vi "sub-select BT device.vi"(8 "error in (no error)":errorcluster, 11 "device list":T1(array[cluster])) -> (0 "error out":errorcluster, 2 "Canceled by user":bool, 3 "Address":string)   [LabVIEW 2016]
doc: "The VI prompts a window that allows the user to select the device and returns the selected device address."
panel:
  in  "Cancel Button":bool
  in  "OK Button":bool
  in  "Select Device":i32(listbox)
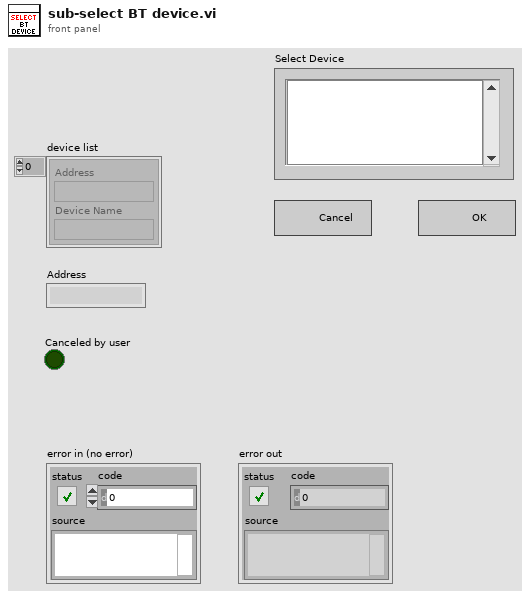
[diagram p1: front panel]
types:
  T1 = cluster{"Address":string, "Device Name":string}[]
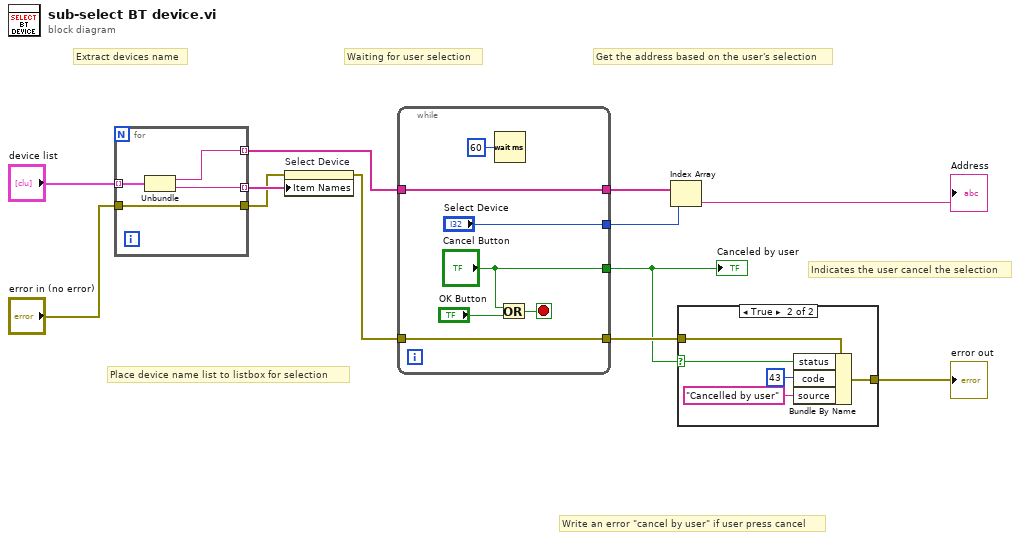
[diagram p0: block diagram]
diagram:
  # "Write an error \"cancel by user\" if user press cancel"
  # "Indicates the user cancel the selection"
  # "Get the address based on the user's selection"
  # "Waiting for user selection"
  # "Place device name list to listbox for selection"
  # "Extract devices name"
  n1 = for {
    tunnel: "device list" -> [w16] mode=indexing
    tunnel: [w15] -> w10 mode=indexing
    tunnel: [w14] -> w11 mode=indexing
    tunnel: [w13] -> w3
    tunnel: "error in (no error)" -> [w13]
    n2 = Unbundle(w16) -> ("Address"=w15:string, "Device Name"=w14:string)
  }
  n3 = property on="Select Device" class="LstBox (strict)"(error in=w3, "Item Names"=w11) -> (error out=w1:errorcluster)  [unwired: 1 in, 1 out]
  n4 = while {
    tunnel: w10 -> [w22]
    tunnel: ["Select Device"] -> w9
    tunnel: [w22] -> w8
    tunnel: ["Cancel Button"] -> w4
    tunnel: [w17] -> w6
    tunnel: w1 -> [w17]
    stop <- w20 stop-if-true
    n5 = Wait (ms)(milliseconds to wait=u32 60) -> ()  [unwired: 1 out]
    n6 = Or(x="Cancel Button", y="OK Button") -> (x .or. y?=w20:bool)
  }
  "Canceled by user" <- w4
  n7 = Index Array(array=w8, index=w9) -> (element=→"Address":string)
  n8 = case shown="True" w4 {
    selector: w4 -> [_ w27]
    tunnel: w6 -> [w24 w29]
    tunnel: [w24 w28] -> w5
    frame False {
    }
    frame True {
      n9 = Bundle By Name(cluster=w29, "status"=w27, "code"=43, "source"="Cancelled by user") -> (w28:errorcluster)
    }
  }
  "error out" <- w5
